vi "Subtract.vi"(0 "A":dbl, 5 "B":dbl) -> (4 "C":dbl)   [LabVIEW 2020]
doc: "This vi is an instance of polymorphic vi which can do subtraction"
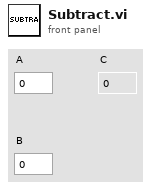
[diagram p1: front panel]
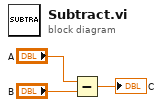
[diagram p0: block diagram]
diagram:
  n1 = Subtract(x="A", y="B") -> (x-y=→"C":dbl)
